vi "TDMS_Property.vi"() -> ()   [LabVIEW 2011]
panel:
  out "property value":i32
  out "found":bool
  out "error out":errorcluster
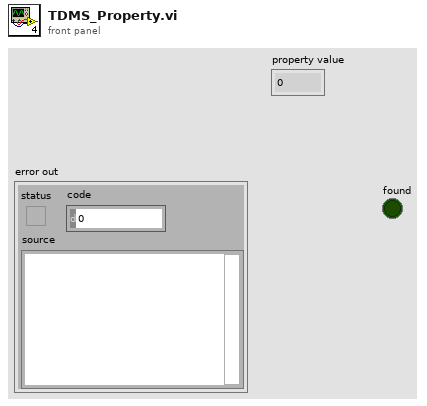
[diagram p1: front panel]
types:
  T1 = enum16{"open", "open or create", "create or replace", "create", "open (read-only)"}
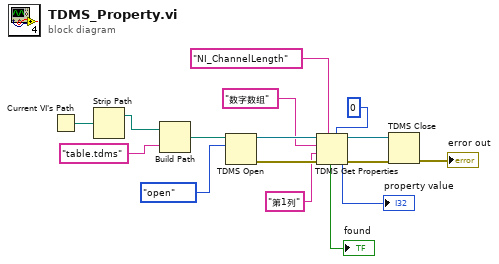
[diagram p0: block diagram]
diagram:
  n1 = Current VI's Path() -> (path=w16:path)
  n2 = Strip Path(path=w16) -> (stripped path=w15:path)  [unwired: 1 out]
  n3 = Build Path(base path=w15, name or relative path="table.tdms") -> (appended path=w10:path)
  n4 = TDMS Open(10:T1."open" ("operation (0:open)"), 11:w10) -> (0:w12:errorcluster, 3:w13:refnum<k34>)  [unwired: 4 in]
  n5 = TDMS Get Properties(5:0, 7:"NI_ChannelLength" ("property name"), 8:w12, 9:"第1列" ("group name"), 10:"数字数组" ("group name"), 11:w13) -> (0:w9:errorcluster, 3:w6:refnum<k34>, 4:→"property value":i32, 6:→"found":bool)  [unwired: 2 out]
  n6 = TDMS Close(8:w9, 11:w6) -> (0:→"error out":errorcluster)  [unwired: 1 out]
